vi "stateTest.vi"() -> ()   [LabVIEW 2010]
uses:
  Statechart 1.lvsc/Inputs.ctl
  Statechart 1.lvsc
  Statechart 1.lvsc/Outputs.ctl
  Statechart 1.lvsc/Trigger.ctl
  <vilib>/Statechart/Infrastructure/RTStatechart/RunTime SCN.xnode
  <vilib>/Statechart/Common/IntGuid.ctl
  <vilib>/Statechart/Common/NI_SC_LVSCCommonFiles.lvlib
  Statechart 1.lvsc/CompanionDiagram.vi/15/SC Main.vi
  <vilib>/Statechart/Common/DbgID.ctl
  <vilib>/sound2/lvsound2.llb/Sound Output Write (DBL Single).vi
  <vilib>/measure/NI_MABase.lvlib
  <vilib>/sound2/lvsound2.llb/Sampling Mode.ctl
  <vilib>/sound2/lvsound2.llb/Sound Data Format.ctl
  <vilib>/DAQmx/write.llb/DAQmx Write (Digital Bool 1Line 1Point).vi
panel:
  in  "DPI":dbl=350.0
  out "Activity monitor":dynamicdata(graph)
  in  "Activity mouse":refnum<visa-resource-name>
  in  "Mouse Axis":bool
  out "Terminate":bool
  in  "stop":bool
  in  "Audio Delay":dbl=4.0
  in  "Shock Duration":dbl=3.0
  in  "Audio Duration":dbl=2.0
  out "Elapsed Time (s)":dbl
  out "Iteration":dbl
  in  "Shock 2":bool
  out "Shock":bool
  out "Audio":bool
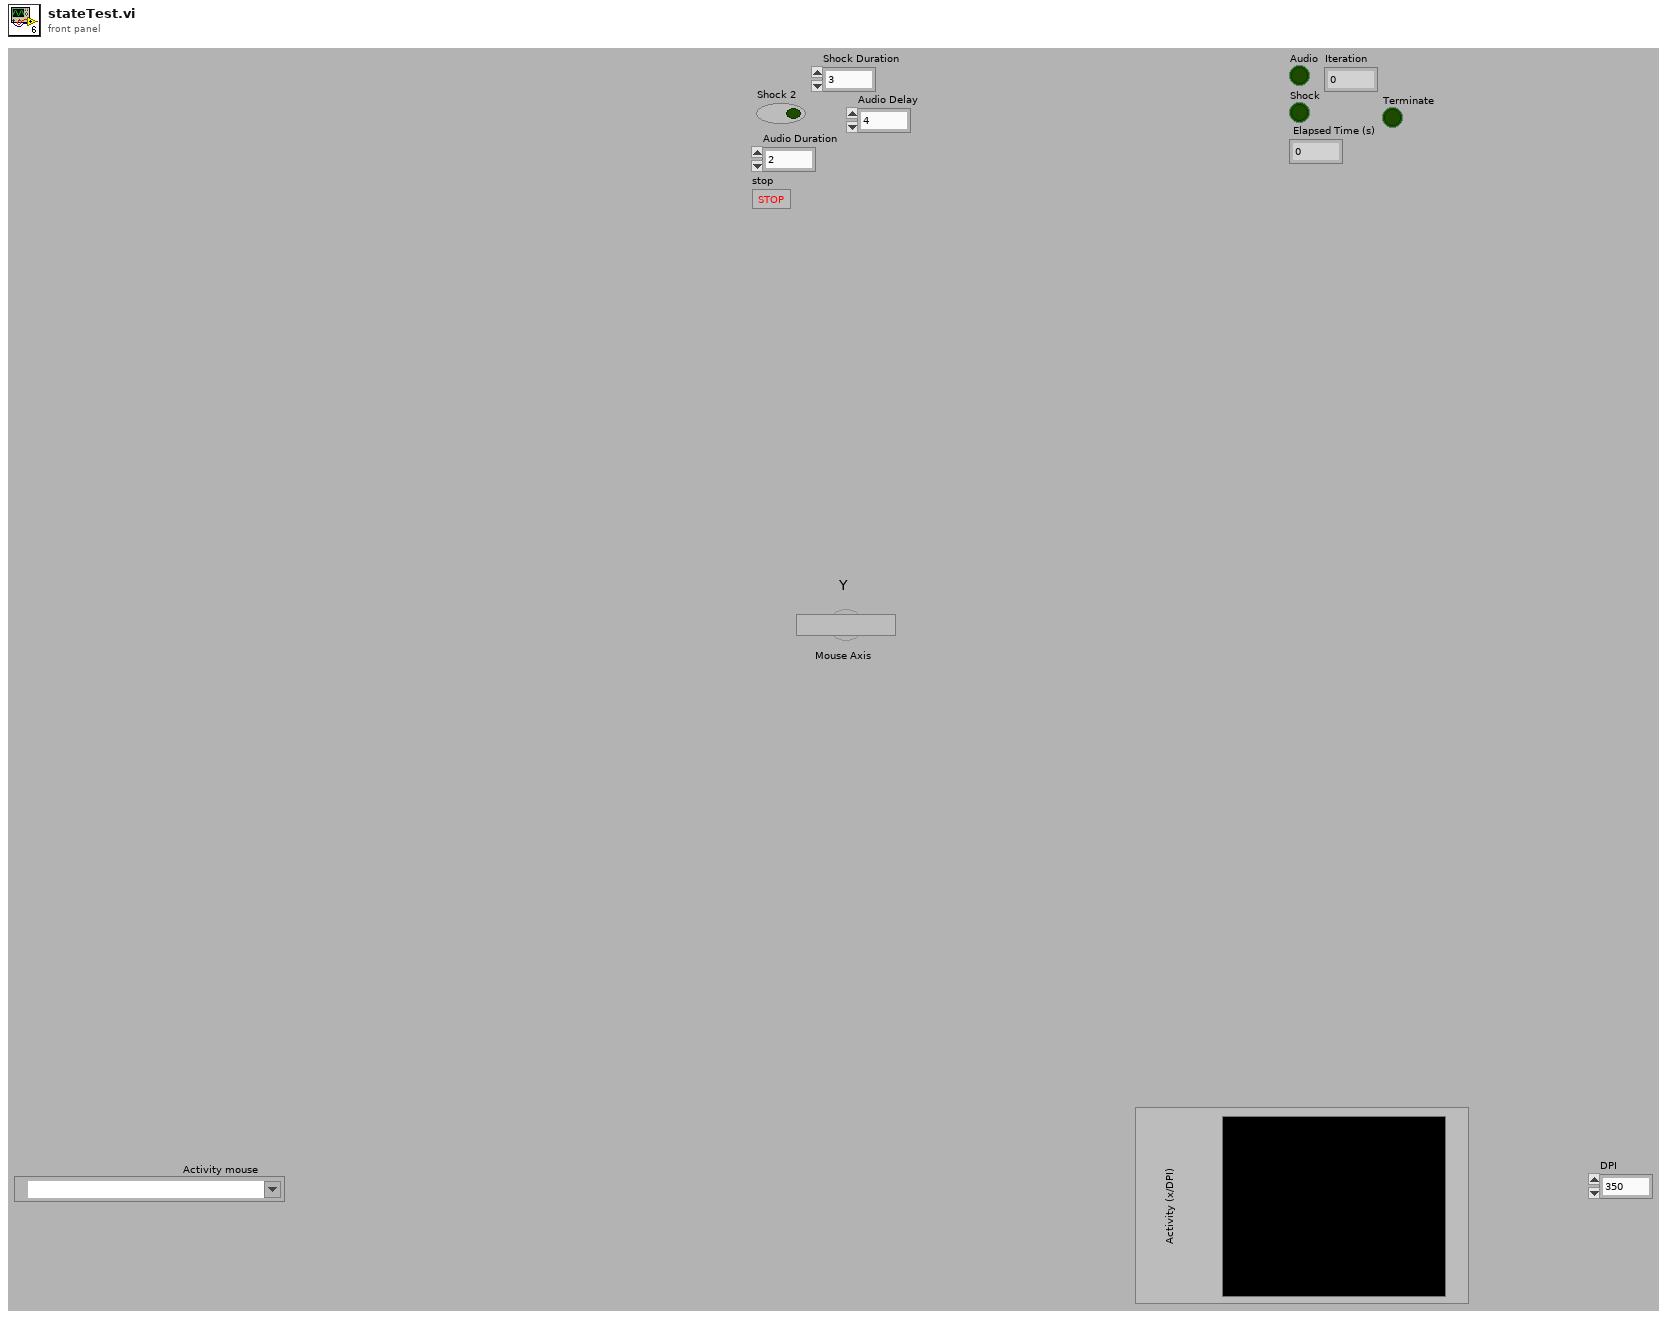
[diagram p1: front panel]
types:
  T1 = typedef "Sound Data Format.ctl" = cluster{"sample rate (S/s)":dbl, "number of channels":i32, "bits per sample":i32}
  T2 = typedef "Sampling Mode.ctl" = i32
  T3 = typedef "Sound Output Task ID.ctl" = u32
  T4 = typedef "Statechart 1.lvsc/Inputs.ctl" = cluster{"Audio Duration":dbl, "Shock Duration ":dbl, "Audio Delay":dbl, "Shock":bool, "timer":dbl, "Iteration":dbl, "Check":dbl}
  T5 = typedef "NI_SC_LVSCCommonFiles.lvlib/IntGuid.ctl" = cluster{"Data1":u32, "Data2":u16, "Data3":u16, "Data4":u8, "Data5":u8, "Data6":u8, "Data11":u8, "Data9":u8, "Data10":u8, "Data8":u8, "Data7":u8}
  T6 = typedef "NI_SC_LVSCCommonFiles.lvlib/DbgID.ctl" = cluster{"VIRef":u32, "IntGUID":T5}
  T7 = typedef "Statechart 1.lvsc/Outputs.ctl" = cluster{"Iteration":dbl, "Audio":bool, "Shock":bool, "Check2":dbl}
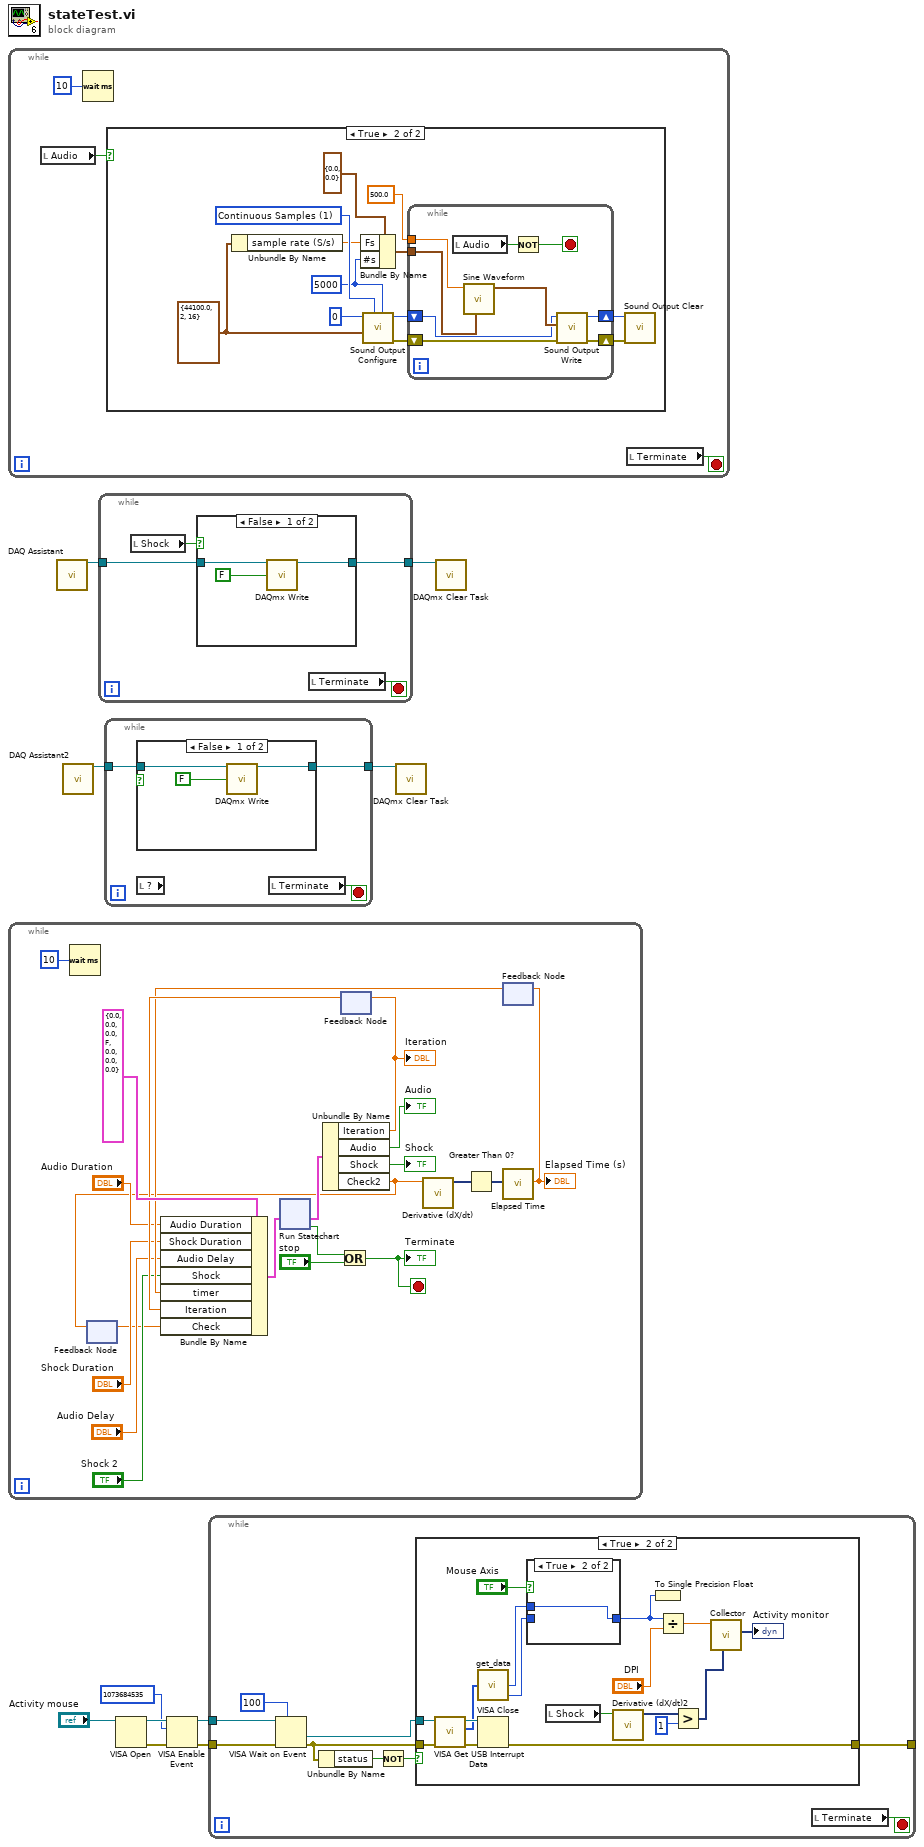
[diagram p0: block diagram]
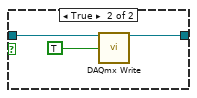
[diagram p4: hidden frame]
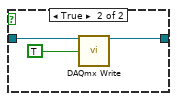
[diagram p5: hidden frame]
diagram:
  n1 = while {
    stop <- w12 stop-if-true
    n2 = local read "Audio"() -> (w13:bool)
    n3 = Wait (ms)(milliseconds to wait=10) -> ()  [unwired: 1 out]
    n4 = case shown="True" w13 {
      frame False {
      }
      frame True {
        w18 = 5000 ("Number of Samples/ch")
        w15 = T1 {"sample rate (S/s)"=44100.0, "number of channels"=2, "bits per sample"=16} ("Sound Format")
        w20 = T2 1 items=["Finite Samples", "Continuous Samples"] ("sample mode")
        n5 = Unbundle By Name(w15) -> ("sample rate (S/s)"=w16:dbl)
        n6 = Bundle By Name(cluster=cluster{"Fs":dbl, "#s":dbl} {"Fs"=0.0, "#s"=0.0} ("sampling info"), "Fs"=w16, "#s"=w18) -> (w17:cluster{"Fs":dbl, "#s":dbl})
        n7 = call <vilib>:"Sound Output Configure.vi"("number of samples/ch"=w18, "sample mode"=w20, "sound format"=w15, "device ID"=u32 0 ("Device ID")) -> ("error out"=w25:errorcluster, "task ID"=w24:T3)  [unwired: 6 in]
        n8 = while {
          shift-right: [w33] -> w23
          shift-left: w25 -> [w29]
          shift-right: [w34] -> w22
          shift-left: w24 -> [w30]
          tunnel: w17 -> [w32]
          tunnel: 500.0 ("Frequency") -> [w28]
          stop <- w26 stop-if-true
          n9 = local read "Audio"() -> (w27:bool)
          n10 = call <vilib>:"Sine Waveform.vi"("sampling info"=w32, "frequency"=w28) -> ("signal out"=w31:waveform(dbl))  [unwired: 8 in, 1 out]
          n11 = Not(x=w27) -> (.not. x?=w26:bool)
          n12 = call-poly <vilib>:"Sound Output Write.vi"("error in (no error)"=w29, "data"=w31, "task ID"=w30) -> ("error out"=w33:errorcluster, "task ID out"=w34:T3)  [unwired: 7 in]
        }
        n13 = call <vilib>:"Sound Output Clear.vi"("error in (no error)"=w23, "task ID"=w22) -> ()  [unwired: 9 in, 1 out]
      }
    }
    n14 = local read "Terminate"() -> (w12:bool)
  }
  n15 = while {
    stop <- w37 stop-if-true
    n16 = Wait (ms)(milliseconds to wait=10) -> ()  [unwired: 1 out]
    n17 = feedback #1() -> (w39:dbl)  [unwired: 1 in]
    n18 = feedback #2() -> (w53:dbl)  [unwired: 1 in]
    n19 = feedback #3() -> (w51:dbl)  [unwired: 1 in]
    n20 = Bundle By Name(cluster=T4 {"Audio Duration"=0.0, "Shock Duration "=0.0, "Audio Delay"=0.0, "Shock"=FALSE, "timer"=0.0, "Iteration"=0.0, "Check"=0.0} ("Inputs"), "Audio Duration"="Audio Duration", "Shock Duration"="Shock Duration", "Audio Delay"="Audio Delay", "Shock"="Shock 2", "timer"=w51, "Iteration"=w53, "Check"=w39) -> (w42:T4)
    n21 = xnode "Run Statechart"("Inputs"=w42) -> ("Terminated?"=w36:bool, "Outputs"=w41:T7)  [unwired: 2 in]
    n22 = Unbundle By Name(w41) -> ("Iteration"=w54:dbl, "Audio"=→"Audio":bool, "Shock"=→"Shock":bool, "Check2"=w38:dbl)
    "Iteration" <- w54
    n23 = feedback-in #1(w38) -> ()
    n24 = Or(x=w36, y="stop") -> (x .or. y?=w37:bool)
    "Terminate" <- w37
    n25 = feedback-in #2(w54) -> ()
    n26 = call "Derivative (dX/dt)"("Signals"=w38) -> ("Result"=w50:dynamicdata)  [unwired: 5 in, 1 out]
    n27 = Greater Than 0?(x=w50) -> (x > 0?=w49:dynamicdata)
    n28 = call "Elapsed Time"("Reset"=w49) -> ("Elapsed Time (s)"=w52:dbl)  [unwired: 11 in, 7 out]
    "Elapsed Time (s)" <- w52
    n29 = feedback-in #3(w52) -> ()
  }
  n30 = call "DAQ Assistant"() -> ("task out"=w10:refnum<k21>)  [unwired: 18 in, 1 out]
  n31 = call "DAQ Assistant2"() -> ("task out"=w8:refnum<k21>)  [unwired: 18 in, 1 out]
  n32 = while {
    tunnel: w10 -> [w76]
    tunnel: [w75] -> w9
    stop <- w73 stop-if-true
    n33 = local read "Shock"() -> (w74:bool)
    n34 = case shown="False" w74 {
      tunnel: w76 -> [w78 w82]
      tunnel: [w77 w80] -> w75
      frame False {
        n35 = call-poly <vilib>:"DAQmx Write.vi"("task/channels in"=w78, "data"=FALSE) -> ("task out"=w77:refnum<k21>)  [unwired: 11 in, 2 out]
      }
      frame True {
        n36 = call-poly <vilib>:"DAQmx Write.vi"("task/channels in"=w82, "data"=TRUE) -> ("task out"=w80:refnum<k21>)  [unwired: 11 in, 2 out]
      }
    }
    n37 = local read "Terminate"() -> (w73:bool)
  }
  n38 = while {
    tunnel: w8 -> [w85]
    tunnel: [w84] -> w7
    stop <- w83 stop-if-true
    n39 = case shown="False" {
      selector: _ -> [_ _]
      tunnel: w85 -> [w87 w91]
      tunnel: [w86 w89] -> w84
      frame False {
        n40 = call-poly <vilib>:"DAQmx Write.vi"("task/channels in"=w87, "data"=FALSE) -> ("task out"=w86:refnum<k21>)  [unwired: 11 in, 2 out]
      }
      frame True {
        n41 = call-poly <vilib>:"DAQmx Write.vi"("task/channels in"=w91, "data"=TRUE) -> ("task out"=w89:refnum<k21>)  [unwired: 11 in, 2 out]
      }
    }
    n42 = local read item#-1() -> ()  [unwired: 1 out]
    n43 = local read "Terminate"() -> (w83:bool)
  }
  n44 = VISA Open(VISA resource name="Activity mouse") -> (VISA resource name=w6:refnum<visa-resource-name>, error out=w5:errorcluster)  [unwired: 1 in, 3 out]
  n45 = VISA Enable Event(8:w5, 10:u32 1073684535 ("event type"), 11:w6) -> (0:w1:errorcluster, 3:w2:refnum<visa-resource-name>)  [unwired: 1 out]
  n46 = while {
    tunnel: w2 -> [w100]
    tunnel: w1 -> [w99]
    tunnel: [w93] -> _
    stop <- w92 stop-if-true
    n47 = VISA Wait on Event(7:u32 100 ("timeout (0)"), 8:w99, 11:w100) -> (0:w94:errorcluster, 1:w95:refnum<visa-resource-name>)  [unwired: 4 out]
    n48 = Unbundle By Name(w94) -> ("status"=w96:bool)
    n49 = Not(x=w96) -> (.not. x?=w97:bool)
    n50 = case shown="True" w97 {
      tunnel: w95 -> [_ w116]
      tunnel: [w101 w115] -> w93
      tunnel: w94 -> [w101 w114]
      frame False {
      }
      frame True {
        n51 = call <vilib>:"VISA Get USB Interrupt Data.vi"("error in (no error)"=w114, "VISA USB Intr Event"=w116) -> ("error out"=w117:errorcluster, "data buffer"=w113:u8[], "VISA USB Intr Event out"=w118:refnum<visa-resource-name>)  [unwired: 7 out]
        n52 = call "get_data.vi"("data buffer"=w113) -> ("X Value"=w111:i8, "Y Value"=w110:i8)  [unwired: 1 out]
        n53 = VISA Close(VISA resource name=w118, error in (no error)=w117) -> (error out=w115:errorcluster)
        n54 = case shown="True" "Mouse Axis" {
          tunnel: w111 -> [_ w120]
          tunnel: [w119 w120] -> w104
          tunnel: w110 -> [w119 _]
          frame False {
          }
          frame True {
          }
        }
        n55 = local read "Shock"() -> (w102:bool)
        n56 = call "Derivative (dX/dt)2"("Signals"=w102) -> ("Result"=w105:dynamicdata)  [unwired: 5 in, 1 out]
        n57 = To Single Precision Float(number=w104) -> ()  [unwired: 1 out]
        n58 = Divide(x=w104, y="DPI") -> (x/y=w107:dbl)
        n59 = Greater?(x=w105, y=1) -> (0:w103:dynamicdata)
        n60 = call "Collector"("Reset"=w103, "Signals"=w107) -> ("Collected Signals"=→"Activity monitor":dynamicdata)  [unwired: 8 in, 1 out]
      }
    }
    n61 = local read "Terminate"() -> (w92:bool)
  }
  n62 = call <vilib>:"DAQmx Clear Task.vi"("task in"=w7) -> ()  [unwired: 14 in, 1 out]
  n63 = call <vilib>:"DAQmx Clear Task.vi"("task in"=w9) -> ()  [unwired: 14 in, 1 out]
